vi "Launch Sub Modules.vi"(8 "error in (no error)":errorcluster, 11 "Executive in":refnum<class "Executive.lvclass">) -> (0 "error out":errorcluster, 3 "Executive out":refnum<class "Executive.lvclass">)   [LabVIEW 2020, in "Executive.lvlib" / "Executive.lvclass"]
uses:
  Executive.lvclass
  C:/Program Files (x86)/National Instruments/LabVIEW 2020/vi.lib/ActorFramework/Actor/Actor.lvclass
  Sub Modules/Chamber Controller/Chamber Controller/Chamber Controller.lvclass
  Sub Modules/Shaker Controller/Shaker Controller/Shaker Controller.lvclass
  Sub Modules/Test Manager/Test Manager/Test Manager.lvclass
  Sub Modules/Web Socket Actor/Web Socket Actor/Web Socket Actor.lvclass
  Executive.lvclass/Executive.ctl
  <vilib>/ActorFramework/Actor/Actor.lvclass
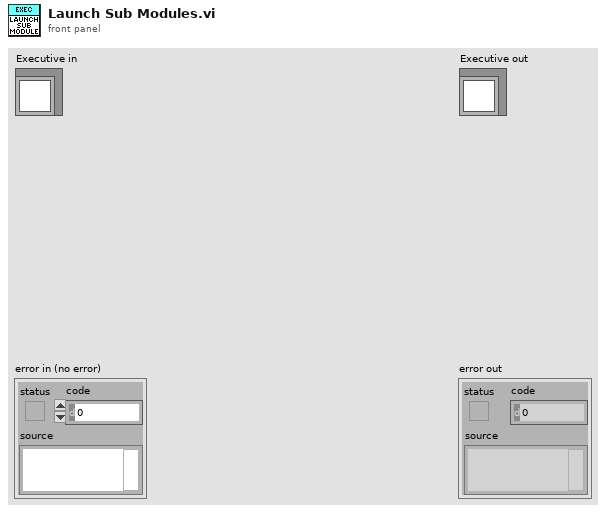
[diagram p1: front panel]
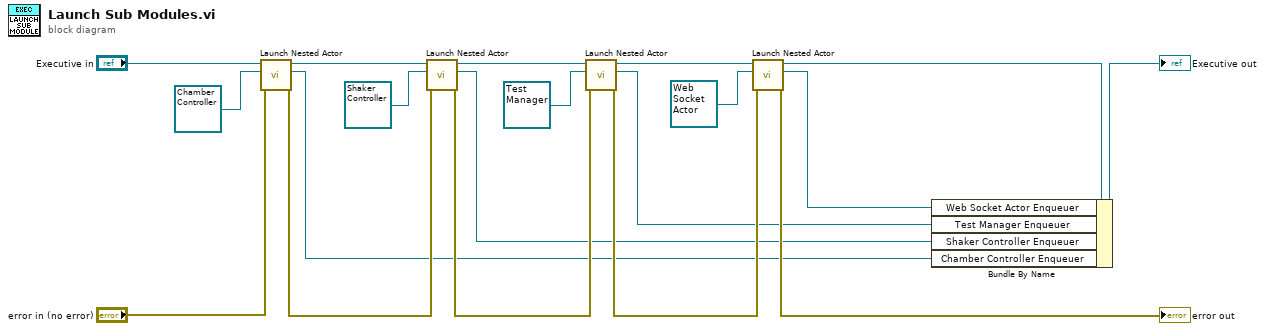
[diagram p0: block diagram]
diagram:
  n1 = call <vilib>:"Launch Nested Actor.vi"("error in (no error)"="error in (no error)", "Nested Actor"=refnum<class "Chamber Controller.lvclass"> refnum ("Chamber Controller.lvlib:Chamber Controller.lvclass"), "Caller Actor in"="Executive in") -> ("error out"=w19:errorcluster, "Nested Actor's Enqueuer"=w5:refnum<class "Message Enqueuer.lvclass">, "Caller Actor out"=w17:refnum<class "Executive.lvclass">)  [unwired: 6 in]
  n2 = call <vilib>:"Launch Nested Actor.vi"("error in (no error)"=w19, "Nested Actor"=refnum<class "Shaker Controller.lvclass"> refnum ("Shaker Controller.lvlib:Shaker Controller.lvclass"), "Caller Actor in"=w17) -> ("error out"=w18:errorcluster, "Nested Actor's Enqueuer"=w4:refnum<class "Message Enqueuer.lvclass">, "Caller Actor out"=w16:refnum<class "Executive.lvclass">)  [unwired: 6 in]
  n3 = call <vilib>:"Launch Nested Actor.vi"("error in (no error)"=w18, "Nested Actor"=refnum<class "Test Manager.lvclass"> refnum ("Test Manager.lvlib:Test Manager.lvclass"), "Caller Actor in"=w16) -> ("error out"=w7:errorcluster, "Nested Actor's Enqueuer"=w3:refnum<class "Message Enqueuer.lvclass">, "Caller Actor out"=w9:refnum<class "Executive.lvclass">)  [unwired: 6 in]
  n4 = call <vilib>:"Launch Nested Actor.vi"("error in (no error)"=w7, "Nested Actor"=refnum<class "Web Socket Actor.lvclass"> refnum ("Web Socket Actor.lvlib:Web Socket Actor.lvclass"), "Caller Actor in"=w9) -> ("error out"=→"error out":errorcluster, "Nested Actor's Enqueuer"=w1:refnum<class "Message Enqueuer.lvclass">, "Caller Actor out"=w8:refnum<class "Executive.lvclass">)  [unwired: 6 in]
  n5 = Bundle By Name(cluster=w8, "Web Socket Actor Enqueuer"=w1, "Test Manager Enqueuer"=w3, "Shaker Controller Enqueuer"=w4, "Chamber Controller Enqueuer"=w5) -> (→"Executive out":refnum<class "Executive.lvclass">)
